vi "am_write.vi"() -> ()   [LabVIEW 2014]
uses:
  aardvark.dll
panel:
  out "Dup Aardvark Handle":i32
  out "Data Written":bool
  in  "Data to Write":u16 format="%.0x"
  out "error out":errorcluster
  in  "Memory ADD":u16=80 max=1023 format="%.0x"
  in  "Address (0x50)":u16=80 max=1023 format="%.0x"
  in  "Aardvark Handle":i32 min=0
  in  "error in (no error)":errorcluster
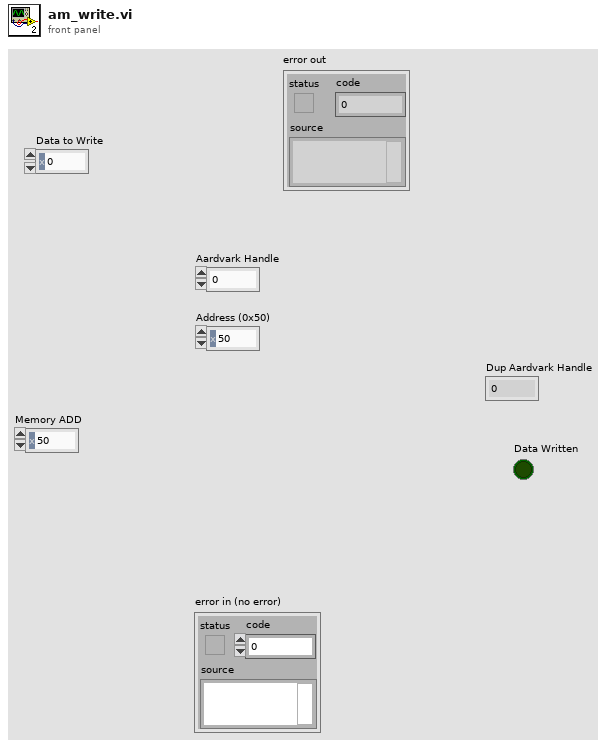
[diagram p1: front panel]
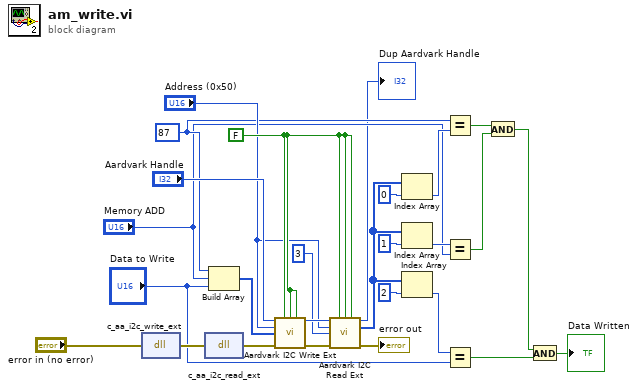
[diagram p0: block diagram]
diagram:
  w22 = FALSE
  w16 = u16 87
  n1 = dll-call lib="aardvark.dll" fn="c_aa_i2c_write_ext"(error in="error in (no error)") -> (error out=w26:errorcluster)  [unwired: 3 in, 1 out]
  n2 = dll-call lib="aardvark.dll" fn="c_aa_i2c_read_ext"(error in=w26) -> (error out=w23:errorcluster)  [unwired: 3 in, 1 out]
  n3 = Build Array(w16, "Memory ADD", "Data to Write") -> (w24:u16[])
  n4 = call <instrlib>:"Aardvark I2C Write Ext.vi"("Aardvark Handle"="Aardvark Handle", "10-bit Addressing? (False)"=w22, "Combined Format? (False)"=w22, "No Stop? (False)"=w22, "Address (0x50)"="Address (0x50)", "Data to Write"=w24, "error in (no error)"=w23) -> ("dup Aardvark Handle"=w21:i32, "error out"=w19:errorcluster)  [unwired: 5 in, 2 out]
  n5 = call <instrlib>:"Aardvark I2C Read Ext.vi"("Aardvark Handle"=w21, "10-bit Addressing? (False)"=w22, "Combined Format? (False)"=w22, "No Stop? (False)"=w22, "Address (0x50)"="Address (0x50)", "Num Bytes to Fetch (64)"=u8 3, "error in (no error)"=w19) -> ("dup Aardvark Handle"=→"Dup Aardvark Handle":i32, "Incoming Data"=w10:u8[], "error out"=→"error out":errorcluster)  [unwired: 5 in, 1 out]
  n6 = Index Array(array=w10, index=0) -> (element=w17:u8)
  n7 = Index Array(array=w10, index=1) -> (element=w13:u8)
  n8 = Index Array(array=w10, index=2) -> (element=w7:u8)
  n9 = Equal?(x=w16, y=w17) -> (x = y?=w12:bool)
  n10 = Equal?(x=w13, y="Memory ADD") -> (x = y?=w11:bool)
  n11 = Equal?(x=w7, y="Data to Write") -> (x = y?=w4:bool)
  n12 = And(x=w12, y=w11) -> (x .and. y?=w8:bool)
  n13 = And(x=w8, y=w4) -> (x .and. y?=→"Data Written":bool)
